vi "byte_stuffing_recod.vi"(3 "String IN":string) -> (0 "bytes added":i32, 1 "String OUT":string, 2 "error out":errorcluster)   [LabVIEW 2010]
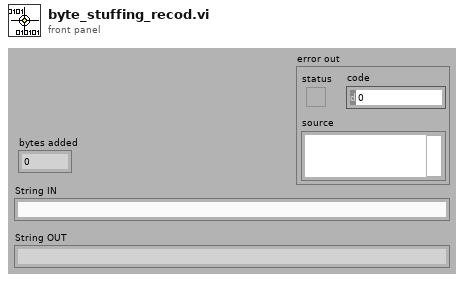
[diagram p1: front panel]
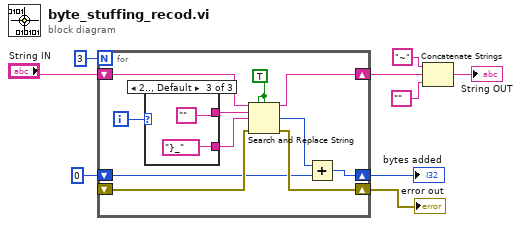
[diagram p0: block diagram]
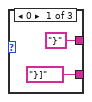
[diagram p2: hidden frame]
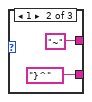
[diagram p3: hidden frame]
diagram:
  n1 = for {
    N: 3 -> [_]
    shift-right: [w18] -> w5
    shift-left: "String IN" -> [w17]
    shift-right: [w15] -> w3
    shift-left: _ -> [w14]
    shift-right: [w11] -> w7
    shift-left: 0 -> [w10]
    i -> [w16]
    w12 = TRUE ("ignore case? (F)")
    n2 = case shown="2.., Default" w16 {
      tunnel: ["}" "~" ""] -> w20
      tunnel: ["}]" "}^" "}_"] -> w19
      frame 0 {
      }
      frame 1 {
      }
      frame 2.., Default {
      }
    }
    n3 = Search and Replace String(replace all?=w12, case sensitive?=w12, input string=w17, search string=w20, replace string=w19, error in=w14) -> (result string=w18:string, number of replacements=w13:i32, error out=w15:errorcluster)  [unwired: 2 in, 1 out]
    n4 = Add(x=w13, y=w10) -> (x+y=w11:i32)
  }
  "bytes added" <- w7
  "error out" <- w3
  n5 = Concatenate Strings("~" ("Lectura 2"), w5, "" ("Lectura 2")) -> (→"String OUT":string)
